vi "Begin LabviewIngestService IngestDataStreamBool.vi"(6 "contextId":T1, 8 "error in":errorcluster, 9 "timeout (ms)":i32=-1, 11 "gRPC ID":T1) -> (0 "error out":errorcluster, 2 "Call Id Out":T1, 3 "gRPC ID out":T1)   [LabVIEW 2024, in "SiftProxy_client.lvlib"]
uses:
  SiftProxy_client.lvlib
  <vilib>/gRPC/LabVIEW gRPC Library/Shared/grpcId.ctl
  <vilib>/gRPC/LabVIEW gRPC Library/grpc-lvsupport-release.lvlib
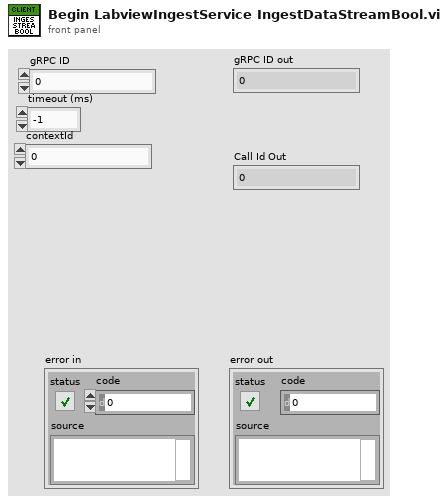
[diagram p1: front panel]
types:
  T1 = typedef "grpc-lvsupport-release.lvlib/grpcId.ctl" = u64
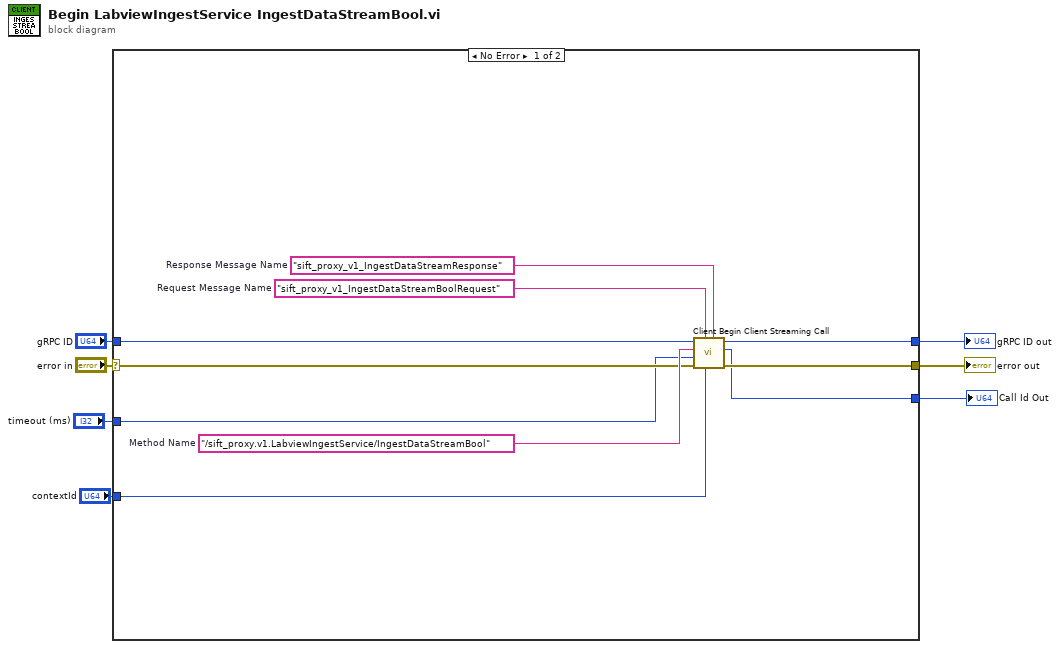
[diagram p0: block diagram]
diagram:
  n1 = case shown="No Error" "error in" {
    selector: "error in" -> [w14 w18]
    tunnel: [w13 w18] -> w6
    tunnel: "gRPC ID" -> [w12 w19]
    tunnel: [w11 w19] -> w4
    tunnel: [w10 _] -> w3
    tunnel: "timeout (ms)" -> [w9 _]
    tunnel: "contextId" -> [w8 _]
    frame No Error {
      w15 = "sift_proxy_v1_IngestDataStreamResponse"  # Response Message Name
      w16 = "sift_proxy_v1_IngestDataStreamBoolRequest"  # Request Message Name
      w17 = "/sift_proxy.v1.LabviewIngestService/IngestDataStreamBool"  # Method Name
      n2 = call <vilib>:"Client Begin Client Streaming Call.vi"("Response Message Name"=w15, "contextId"=w8, "Request Message Name"=w16, "error in"=w14, "timeout (ms)"=w9, "Method Name"=w17, "ClientID in"=w12) -> ("error out"=w13:errorcluster, "Call ID out"=w10:T1, "ClientID out"=w11:T1)  [unwired: 2 in]
    }
    frame Error {
    }
  }
  "error out" <- w6
  "gRPC ID out" <- w4
  "Call Id Out" <- w3
